vi "FVIR UI Setup Part 1.vi"(8 "error in (no error)":errorcluster, 10 "Initialize? in":bool, 11 "Queue in":refnum<queue>) -> (0 "error out":errorcluster, 3 "Queue out":refnum<queue>)   [LabVIEW 2020]
uses:
  Message Queue/Message Cluster.ctl
  Message Queue/Enqueue Message (Single).vi
  Message Queue/Message Queue.lvlib
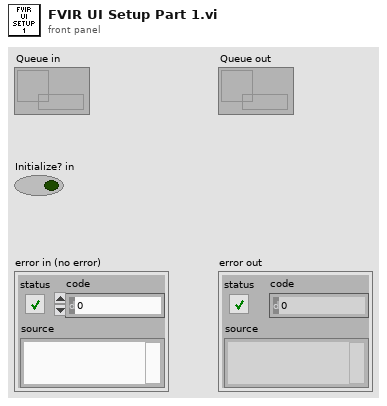
[diagram p1: front panel]
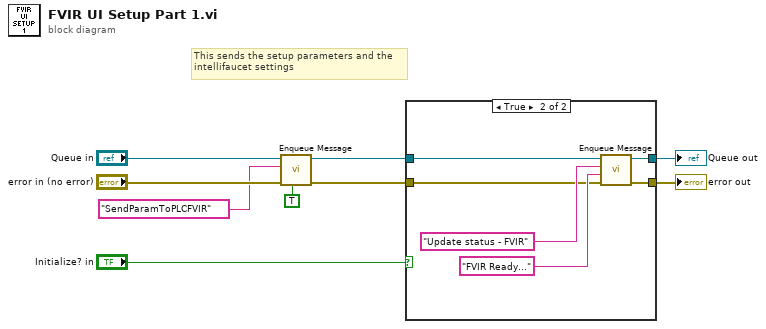
[diagram p0: block diagram]
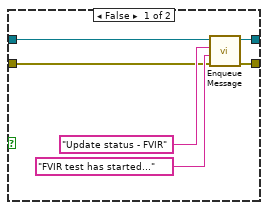
[diagram p2: hidden frame]
diagram:
  # "This sends the setup parameters and the\nintellifaucet settings"
  n1 = call-poly "Enqueue Message.vi"("Priority Message? (F)"=TRUE, "error in (no error)"="error in (no error)", "Message"="SendParamToPLCFVIR" ("Acquiring and Logging..."), "Message Queue"="Queue in") -> ("error out"=w5:errorcluster, "dup Message Queue"=w6:refnum<queue>)  [unwired: 6 in]
  n2 = case shown="True" "Initialize? in" {
    tunnel: w5 -> [w11 w19]
    tunnel: w6 -> [w13 w18]
    tunnel: [w10 w17] -> w9
    tunnel: [w12 w16] -> w7
    frame False {
      n3 = call-poly "Enqueue Message.vi"("error in (no error)"=w11, "Message Data"="FVIR test has started..." ("Acquiring and Logging..."), "Message"="Update status - FVIR", "Message Queue"=w13) -> ("error out"=w10:errorcluster, "dup Message Queue"=w12:refnum<queue>)  [unwired: 6 in]
    }
    frame True {
      n4 = call-poly "Enqueue Message.vi"("error in (no error)"=w19, "Message Data"="FVIR Ready..." ("Ready..."), "Message"="Update status - FVIR", "Message Queue"=w18) -> ("error out"=w17:errorcluster, "dup Message Queue"=w16:refnum<queue>)  [unwired: 6 in]
    }
  }
  "error out" <- w9
  "Queue out" <- w7
